vi "Read files ALL(Recorder).vi"(11 "Path":path) -> (0 "Table 2":string[][](table), 1 "Table":string[][](table), 2 "Graph 2":dynamicdata(graph), 3 "Graph":dynamicdata(graph))   [LabVIEW 2020, in "GPP.lvlib"]
uses:
  GPP.lvlib
panel:
  out "CURRENT 2":dbl[](array[numeric])
  out "C 2":dbl
  out "VOLTAGE 2":dbl[](array[numeric])
  out "V 2":dbl
  out "VOLTAGE":dbl[](array[numeric])
  out "CURRENT":dbl[](array[numeric])
  out "V":dbl
  out "C":dbl
  out "N":dbl
  out "NUMBER":dbl[](array[numeric])
  # "CH1"
  # "CH2"
  # "CH1"
  # "CH2"
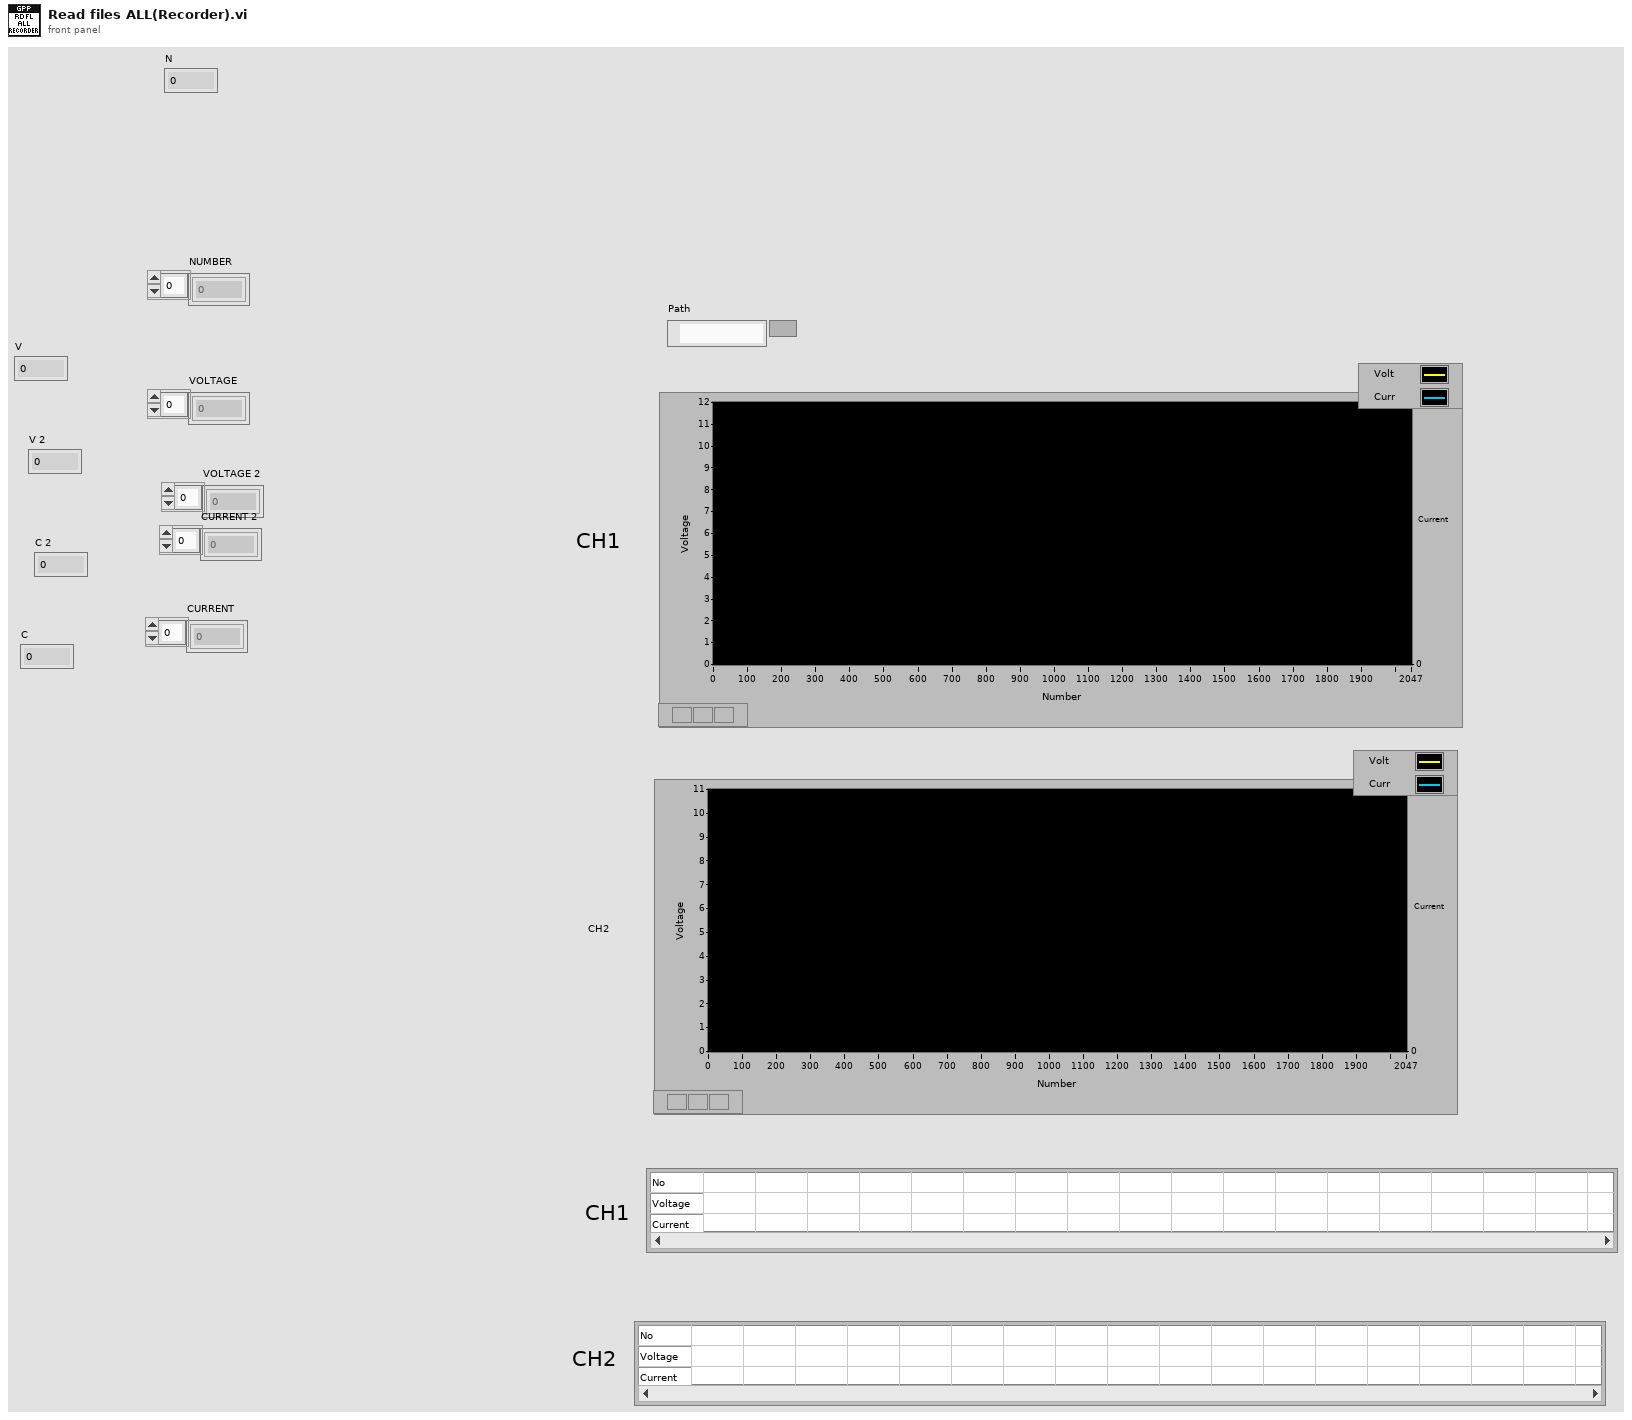
[diagram p1: front panel]
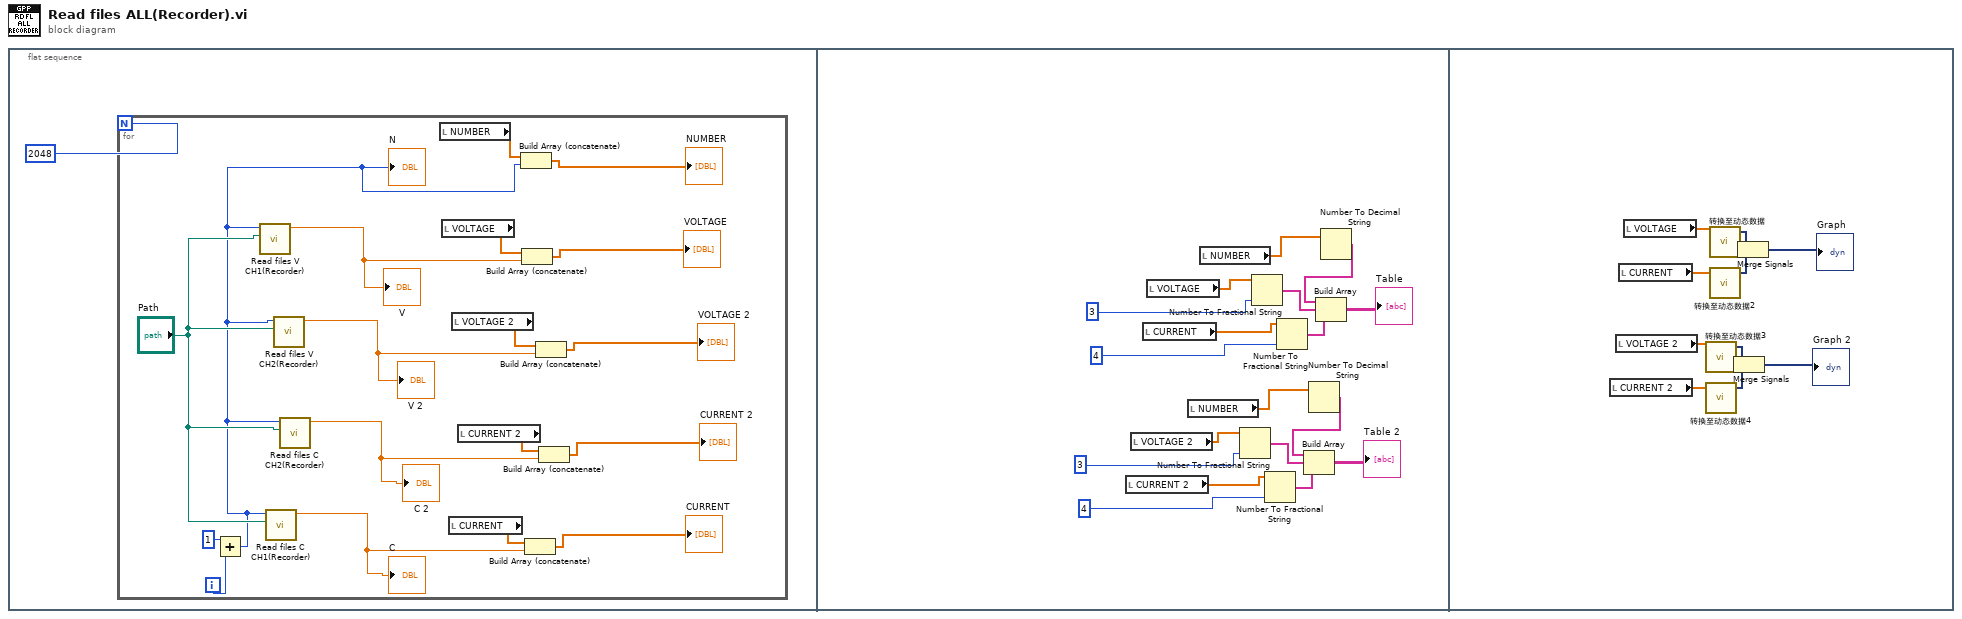
[diagram p0: block diagram]
diagram:
  n1 = flat-sequence {
    frame #0 {
      n2 = for {
        N: 2048 -> [_]
        i -> [w13]
        n3 = Add(x=1, y=w13) -> (x+y=w2:i32)
        "N" <- w2
        n4 = call "Read files V CH1(Recorder).vi"("Path"="Path", "Number"=w2) -> ("Voltage"=w19:dbl)  [unwired: 9 in]
        "V" <- w19
        n5 = call "Read files C CH1(Recorder).vi"("Path"="Path", "Number"=w2) -> ("Current"=w18:dbl)  [unwired: 9 in]
        "C" <- w18
        n6 = call "Read files V CH2(Recorder).vi"("Path"="Path", "Number"=w2) -> ("Voltage"=w7:dbl)  [unwired: 9 in]
        "V 2" <- w7
        n7 = call "Read files C CH2(Recorder).vi"("Path"="Path", "Number"=w2) -> ("Current"=w4:dbl)  [unwired: 9 in]
        "C 2" <- w4
        n8 = local read "NUMBER"() -> (w11:dbl[])
        n9 = local read "VOLTAGE"() -> (w17:dbl[])
        n10 = local read "CURRENT"() -> (w16:dbl[])
        n11 = local read "VOLTAGE 2"() -> (w8:dbl[])
        n12 = local read "CURRENT 2"() -> (w5:dbl[])
        n13 = Build Array (concatenate)(w11, w2) -> (→"NUMBER":dbl[])
        n14 = Build Array (concatenate)(w17, w19) -> (→"VOLTAGE":dbl[])
        n15 = Build Array (concatenate)(w16, w18) -> (→"CURRENT":dbl[])
        n16 = Build Array (concatenate)(w8, w7) -> (→"VOLTAGE 2":dbl[])
        n17 = Build Array (concatenate)(w5, w4) -> (→"CURRENT 2":dbl[])
      }
    }
    frame #1 {
      n18 = local read "CURRENT 2"() -> (w20:dbl[])
      n19 = local read "VOLTAGE 2"() -> (w25:dbl[])
      n20 = local read "CURRENT"() -> (w37:dbl[])
      n21 = local read "VOLTAGE"() -> (w32:dbl[])
      n22 = local read "NUMBER"() -> (w24:dbl[])
      n23 = local read "NUMBER"() -> (w33:dbl[])
      n24 = Number To Fractional String(number=w25, precision (6)=3) -> (F-format string=w26:string[])  [unwired: 2 in]
      n25 = Number To Fractional String(number=w32, precision (6)=3) -> (F-format string=w31:string[])  [unwired: 2 in]
      n26 = Number To Fractional String(number=w20, precision (6)=4) -> (F-format string=w21:string[])  [unwired: 2 in]
      n27 = Number To Fractional String(number=w37, precision (6)=4) -> (F-format string=w36:string[])  [unwired: 2 in]
      n28 = Number To Decimal String(number=w24) -> (decimal integer string=w22:string[])  [unwired: 1 in]
      n29 = Build Array(w22, w26, w21) -> (→"Table 2":string[][])
      n30 = Number To Decimal String(number=w33) -> (decimal integer string=w35:string[])  [unwired: 1 in]
      n31 = Build Array(w35, w31, w36) -> (→"Table":string[][])
    }
    frame #2 {
      n32 = local read "CURRENT 2"() -> (w38:dbl[])
      n33 = local read "VOLTAGE 2"() -> (w39:dbl[])
      n34 = local read "CURRENT"() -> (w47:dbl[])
      n35 = local read "VOLTAGE"() -> (w46:dbl[])
      n36 = call "转换至动态数据3"("Array"=w39) -> ("Dynamic Data Type"=w40:dynamicdata)  [unwired: 3 in]
      n37 = call "转换至动态数据4"("Array"=w38) -> ("Dynamic Data Type"=w41:dynamicdata)  [unwired: 3 in]
      n38 = call "转换至动态数据"("Array"=w46) -> ("Dynamic Data Type"=w45:dynamicdata)  [unwired: 3 in]
      n39 = call "转换至动态数据2"("Array"=w47) -> ("Dynamic Data Type"=w44:dynamicdata)  [unwired: 3 in]
      n40 = Merge Signals(w40, w41) -> (→"Graph 2":dynamicdata)
      n41 = Merge Signals(w45, w44) -> (→"Graph":dynamicdata)
    }
  }
